vi "Read ConflictHandler.vi"(8 "error in (no error)":errorcluster, 11 "ParserConfig in":refnum<class "ParserConfig.lvclass">) -> (0 "error out":errorcluster, 2 "ConflictHandler":string="error", 3 "ParserConfig out":refnum<class "ParserConfig.lvclass">)   [LabVIEW 2022 SP3, in "ArgumentParser.lvlib" / "ParserConfig.lvclass"]
uses:
  ParserConfig.lvclass
  ParserConfig.lvclass/ParserConfig.ctl
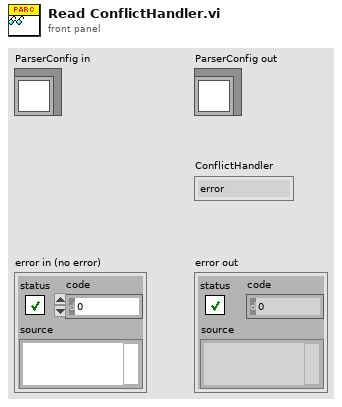
[diagram p1: front panel]
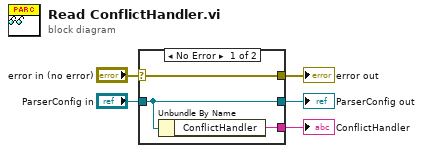
[diagram p0: block diagram]
diagram:
  n1 = case shown="No Error" "error in (no error)" {
    selector: "error in (no error)" -> [w8 w9]
    tunnel: [w8 w9] -> w4
    tunnel: [w7 w10] -> w2
    tunnel: "ParserConfig in" -> [w7 w10]
    tunnel: [w6 _] -> w1
    frame No Error {
      n2 = Unbundle By Name(w7) -> ("ConflictHandler"=w6:string)
    }
    frame Error {
    }
  }
  "error out" <- w4
  "ParserConfig out" <- w2
  "ConflictHandler" <- w1
